vi "LIMITSWITCHREAD.vi"   [LabVIEW 2014]
uses:
  limitSwitchGlobals.vi
types:
  T1 = typedef "WPI_DigitalInputDevRef.ctl" = cluster{"DevStatus":errorcluster, "DIO Channel":T2, "Controller":T3}
  T2 = typedef "FPGA_DIOChannel.ctl" = enum8{"DIO 0", "DIO 1", "DIO 2", "DIO 3", "DIO 4", "DIO 5", "DIO 6", "DIO 7", "DIO 8", "DIO 9", "DIO MXP 0", "DIO MXP 1", "DIO MXP 2", "DIO MXP 3", "DIO MXP 4", "DIO MXP 5", "DIO MXP 6", "DIO MXP 7", "DIO MXP 8", "DIO MXP 9", "DIO MXP 10", "DIO MXP 11", "DIO MXP 12", "DIO MXP 13", "DIO MXP 14", "DIO MXP 15", "Invalid"}
  T3 = typedef "FPGA_TypedefDigitalModule.ctl" = enum16{"Controller 1"}
  T4 = typedef "WPI_EncoderDevRef.ctl" = cluster{"DevStatus":errorcluster, "EncoderIndex":T5, "CounterIndex":T6, "DistancePerCount":dbl, "Decoding Type":T7}
  T5 = typedef "FPGA_EncoderIdx.ctl" = enum8{"Enc 0", "Enc 1", "Enc 2", "Enc 3", "Enc 4", "Enc 5", "Enc 6", "Enc 7", "Invalid"}
  T6 = typedef "FPGA_CounterCtrSystemIndex.ctl" = enum8{"Ctr 0", "Ctr 1", "Ctr 2", "Ctr 3", "Ctr 4", "Ctr 5", "Ctr 6", "Ctr 7", "Invalid"}
  T7 = typedef "WPI_EncoderType.ctl" = enum16{"1x", "2x", "4x"}
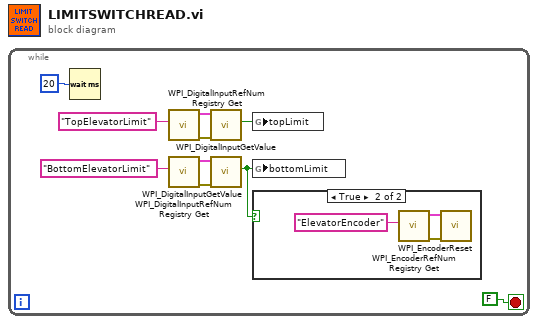
[diagram p0: block diagram]
diagram:
  n1 = while {
    stop <- FALSE stop-if-true
    n2 = Wait (ms)(milliseconds to wait=u32 20) -> ()  [unwired: 1 out]
    n3 = call <vilib>:"WPI_DigitalInputRefNum Registry Get.vi"("refnum name"="TopElevatorLimit") -> ("error out"=w7:errorcluster, "DigitalInputDevRef"=w8:T1)  [unwired: 9 in]
    n4 = call <vilib>:"WPI_DigitalInputRefNum Registry Get.vi"("refnum name"="BottomElevatorLimit") -> ("error out"=w5:errorcluster, "DigitalInputDevRef"=w6:T1)  [unwired: 9 in]
    n5 = call <vilib>:"WPI_DigitalInputGetValue.vi"("error in (no error)"=w7, "DigitalInputDevRef"=w8) -> ("Value"=w4:bool)  [unwired: 7 in, 2 out]
    n6 = call <vilib>:"WPI_DigitalInputGetValue.vi"("error in (no error)"=w5, "DigitalInputDevRef"=w6) -> ("Value"=w1:bool)  [unwired: 7 in, 2 out]
    n7 = global write "limitSwitchGlobals.vi" "topLimit"(w4) -> ()
    n8 = global write "limitSwitchGlobals.vi" "bottomLimit"(w1) -> ()
    n9 = case shown="True" w1 {
      frame False {
      }
      frame True {
        n10 = call <vilib>:"WPI_EncoderRefNum Registry Get.vi"("refnum name"="ElevatorEncoder") -> ("error out"=w11:errorcluster, "EncoderDevRef"=w12:T4)  [unwired: 9 in]
        n11 = call <vilib>:"WPI_EncoderReset.vi"("error in (no error)"=w11, "EncoderDevRef"=w12) -> ()  [unwired: 8 in, 2 out]
      }
    }
  }
